vi "Module Add.vi"(7 "Parent ID":i32, 8 "error in (no error)":errorcluster, 9 "Config Section":string, 10 "Config Path":path, 11 "Name":string) -> (0 "error out":errorcluster, 3 "Module":T1)   [LabVIEW 2018, in "Core.lvlib"]
uses:
  Core.lvlib
  Controls/Module Instance.ctl
  Controls/Module.ctl
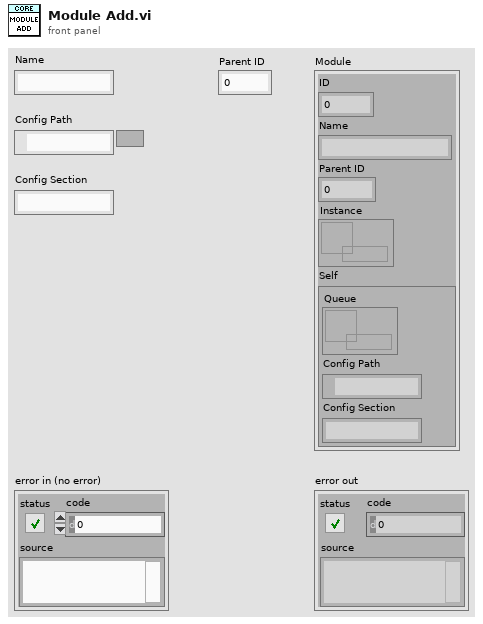
[diagram p1: front panel]
types:
  T1 = typedef "Core.lvlib/Module.ctl" = cluster{"ID":i32, "Name":string, "Parent ID":i32, "Instance":refnum<data-value>, "Self":T2}
  T2 = typedef "Core.lvlib/Module Instance.ctl" = cluster{"Queue":refnum<queue>, "Config Path":path, "Config Section":string}
  T3 = cluster{"ID":i32, "Name":string, "Parent ID":i32, "Instance":refnum<data-value>}[]
  T4 = cluster{"ID":i32, "Name":string, "Parent ID":i32, "Instance":refnum<data-value>}
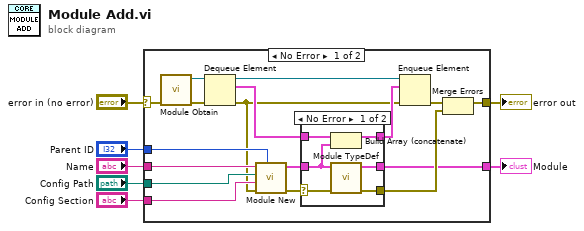
[diagram p0: block diagram]
diagram:
  n1 = case shown="No Error" "error in (no error)" {
    selector: "error in (no error)" -> [w24 w33]
    tunnel: [w12 w33] -> w6
    tunnel: "Parent ID" -> [w17 _]
    tunnel: "Name" -> [w16 _]
    tunnel: "Config Path" -> [w15 _]
    tunnel: "Config Section" -> [w14 _]
    tunnel: [w8 _] -> w1
    frame No Error {
      n2 = call "Module Obtain.vi"("error in (no error)"=w24) -> ("error out"=w23:errorcluster, "Modules"=w22:refnum<queue>)  [unwired: 8 in, 1 out]
      n3 = Dequeue Element(queue=w22, error in (no error)=w23) -> (queue out=w20:refnum<queue>, element=w19:T3, error out=w11:errorcluster)  [unwired: 1 in, 1 out]
      n4 = call "Module New.vi"("Parent ID"=w17, "error in (no error)"=w11, "Config Section"=w14, "Config Path"=w15, "Name"=w16) -> ("error out"=w10:errorcluster, "Module"=w13:T4)  [unwired: 5 in]
      n5 = case shown="No Error" w10 {
        selector: w10 -> [w28 w31]
        tunnel: w19 -> [w30 w32]
        tunnel: [w29 w32] -> w18
        tunnel: w13 -> [w26 _]
        tunnel: [w27 w31] -> w9
        tunnel: [w25 _] -> w8
        frame No Error {
          n6 = Build Array (concatenate)(w30, w26) -> (w29:T3)
          n7 = call "Module TypeDef.vi"("error in (no error)"=w28, "Module in"=w26) -> ("error out"=w27:errorcluster, "Module"=w25:T1)  [unwired: 8 in]
        }
        frame Error {
        }
      }
      n8 = Enqueue Element(queue=w20, element=w18, error in (no error)=w11) -> (error out=w21:errorcluster)  [unwired: 1 in, 2 out]
      n9 = Merge Errors(w21, w9) -> (w12:errorcluster)
    }
    frame Error {
    }
  }
  "error out" <- w6
  "Module" <- w1
